vi "Convert_ERDs_Brass.vi"(0 "New Header?":bool, 7 "Array":T7[](array[typedef]) {"ERD Number" format="%.0x"}, 11 "Error In":errorcluster) -> (4 "All_ERD_Data_Bundled_Brass":T1, 15 "Error Out":errorcluster)   [LabVIEW 2016]
doc: "This VI parses the data from ERDs in correct format, units, etc. It handles all hex to dec conversions, hex to enum, and hex to boolean conversions.\n\nIf Raw Data from ERD is blank string, then it will output values from shift register."
uses:
  Common/LabVIEW GEA2 Toolkit/LabVIEW_GEA2_Toolkit.lvlibp/type defs/ERD Read Data Out.ctl
  type defs2/All_Bundled_Data_Brass.ctl
  Laundry Tool 1.0 Support/type defs/Version.ctl
  type defs2/ERD_Always_Show_Brass.ctl
  type defs2/CSV_File_String_Arrays.ctl
  type defs2/Fault Table Array.ctl
  Laundry Tool 1.0 Support/type defs/Fault_Table_Info.ctl
  Common/LabVIEW GEA2 Toolkit/LabVIEW_GEA2_Toolkit.lvlibp
panel:
  # "Software Version"
  # "UI"
  # "MC"
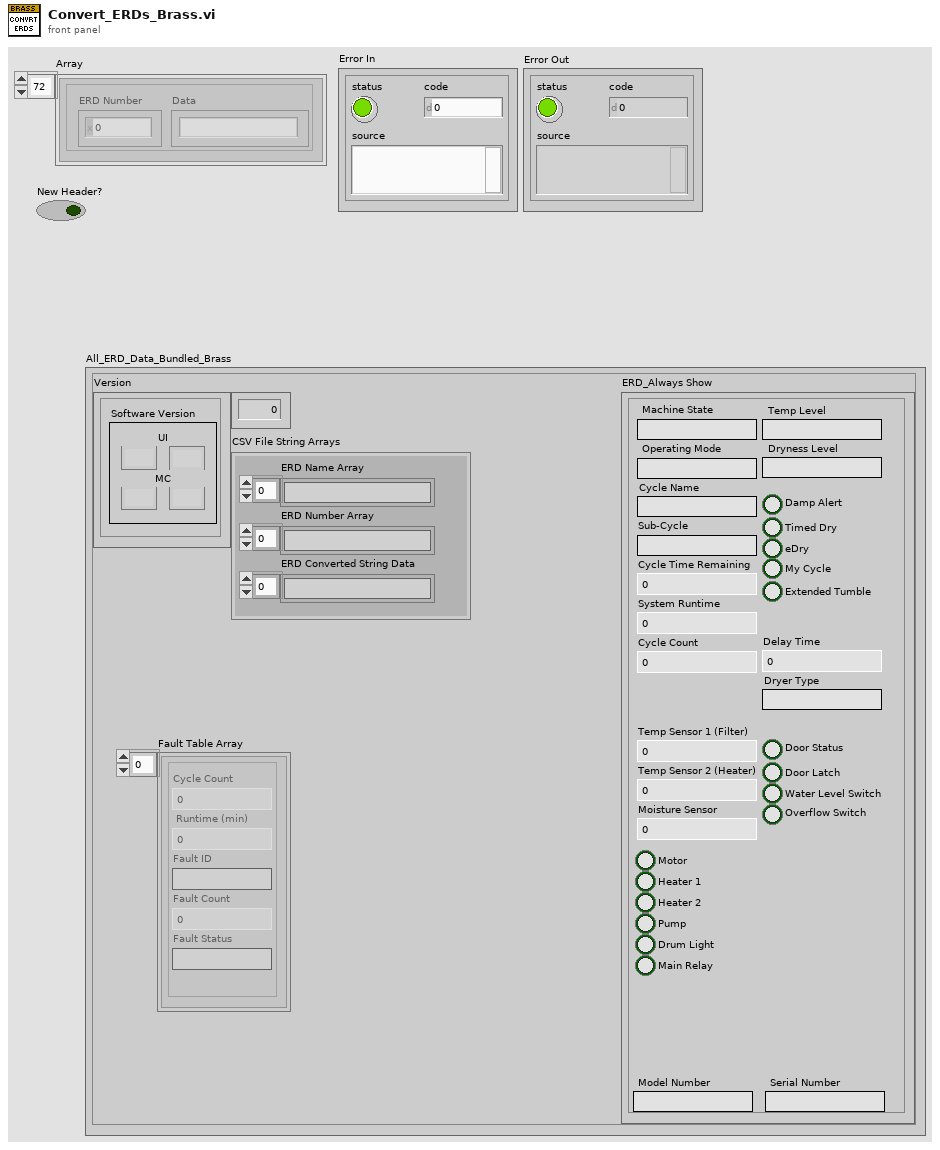
[diagram p1: front panel]
types:
  T1 = typedef "All_Bundled_Data_Brass.ctl" = cluster{"Version":T2, "ERD_Always Show":T3, "Personality Set":u8, "CSV File String Arrays":T4, "Fault Table Array ":T5}
  T2 = typedef "Version.ctl" = cluster{"Critical Major":string, "Critical Minor":string, "Non-Critical Minor":string, "Non-Critical Major":string}
  T3 = typedef "ERD_Always_Show_Brass.ctl" = cluster{"Machine State":string, "Cycle Count":u32, "Dryness Level":string, "Temp Level":string, "Delay Time":u16, "Sub-Cycle":string, "Cycle Name":string, "Model Number":string, "Serial Number":string, "System Runtime":u32, "Cycle Time Remaining":u16, "Operating Mode":string, "Temp Sensor 1 (Filter)":u16, "Water Level Switch":bool, "Overflow Switch":bool, "Door Status":bool, "Door Latch":bool, "Heater 1":bool, "Temp Sensor 2 (Heater)":u16, "Moisture Sensor":u16, "Dryer Type":string, "eDry":bool, "Damp Alert":bool, "Timed Dry":bool, "My Cycle":bool, "Extended Tumble":bool, "Heater 2":bool, "Pump":bool, "Drum Light":bool, "Main Relay":bool, "Motor":bool}
  T4 = typedef "CSV_File_String_Arrays.ctl" = cluster{"ERD Number Array":string[], "ERD Name Array":string[], "ERD Converted String Data":string[]}
  T5 = typedef "Fault Table Array.ctl" = T6[]
  T6 = typedef "Fault_Table_Info.ctl" = cluster{"Cycle Count":u32, " Runtime (min) ":u32, "Fault Status":string, "Fault ID":string, "Fault Count":u16}
  T7 = typedef "LabVIEW_GEA2_Toolkit.lvlibp/ERD Read Data Out.ctl" = cluster{"ERD Number":u16, "Data":string}
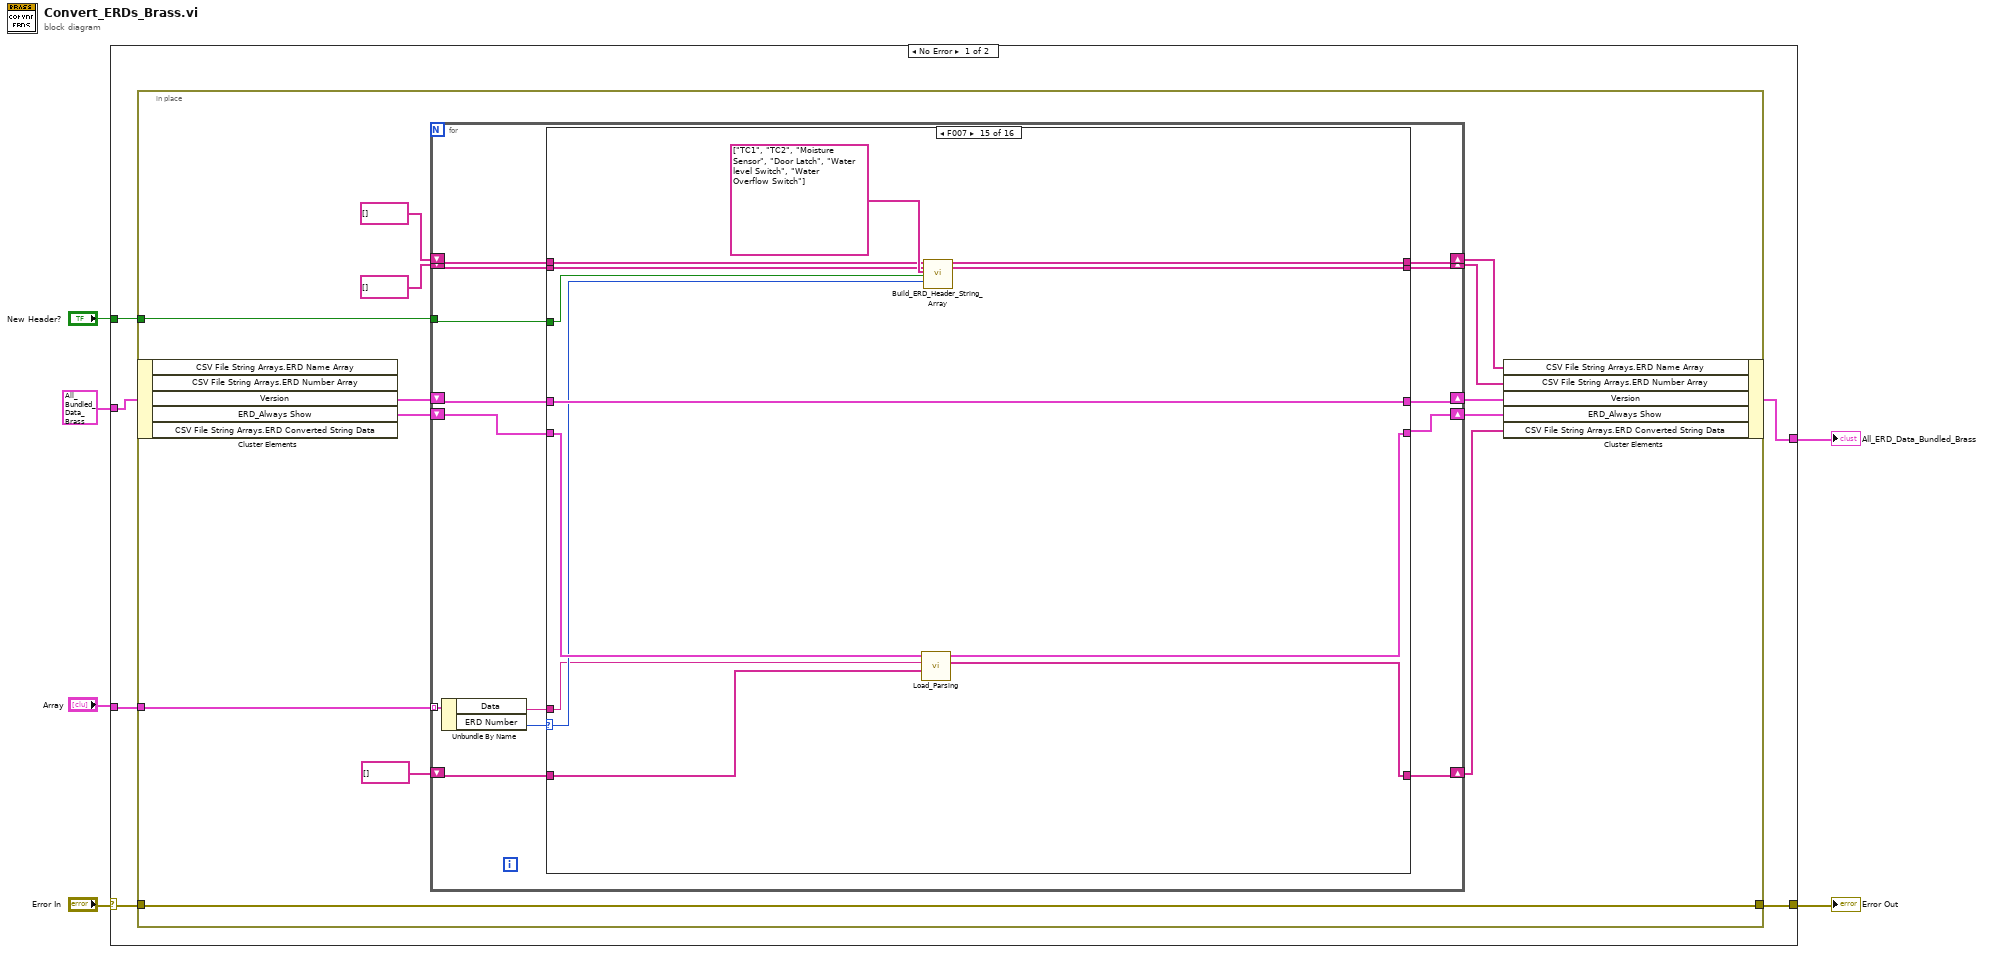
[diagram p0: block diagram]
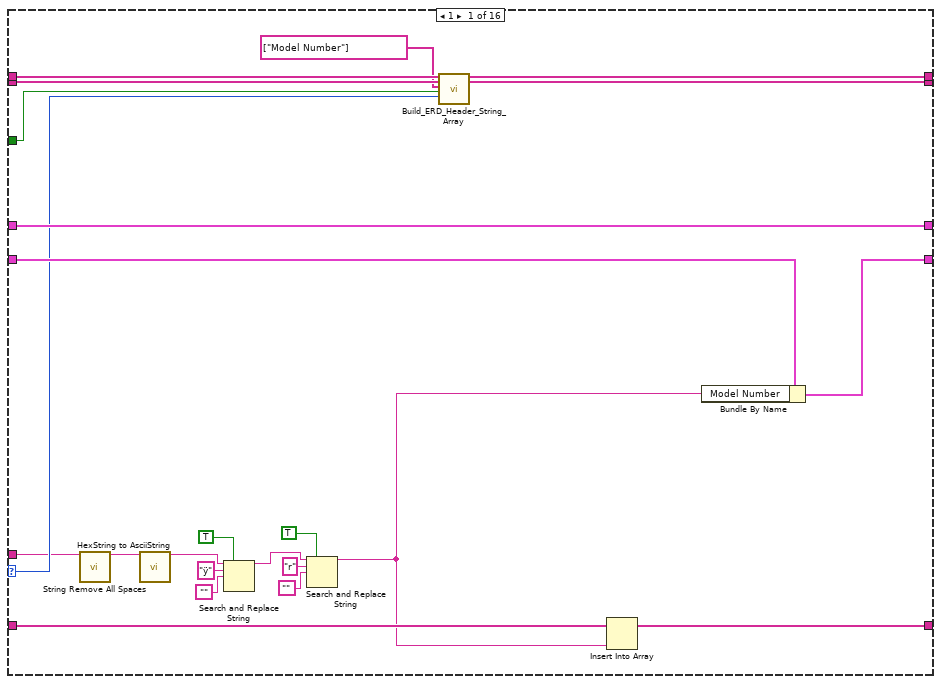
[diagram p2: hidden frame]
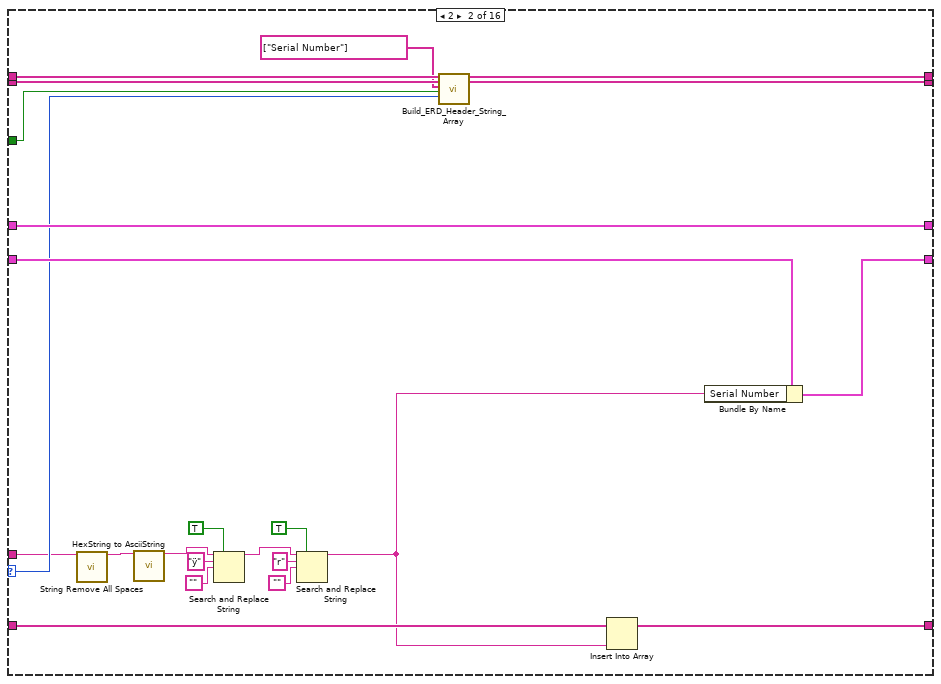
[diagram p3: hidden frame]
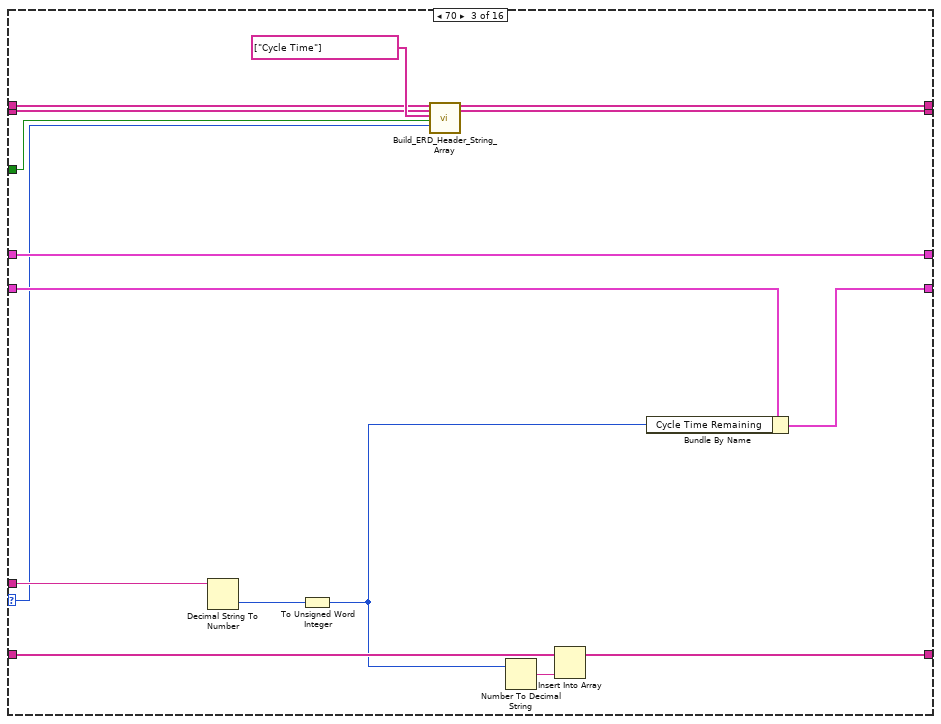
[diagram p4: hidden frame]
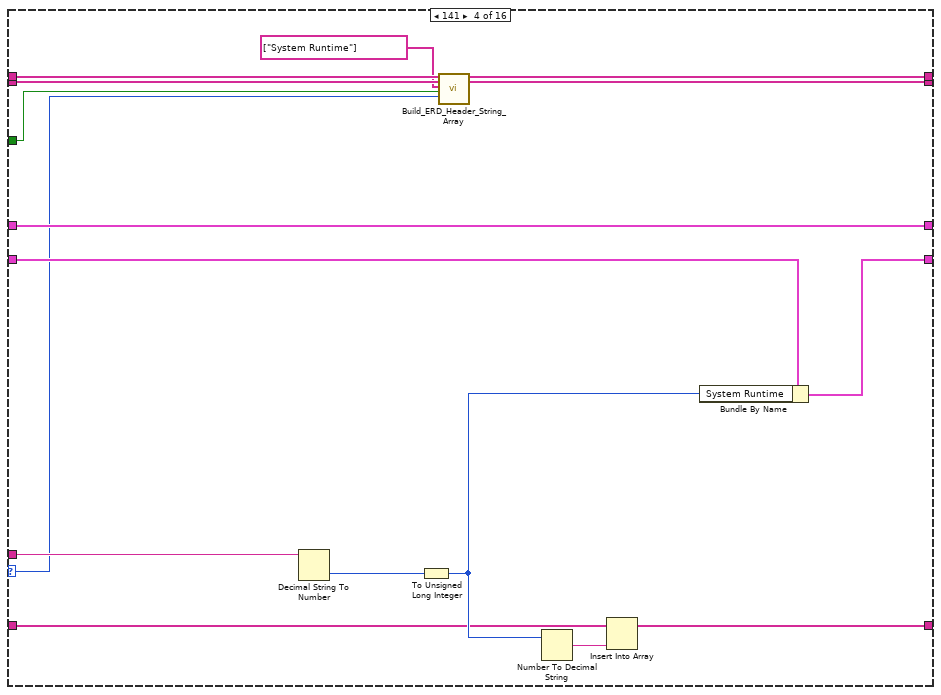
[diagram p5: hidden frame]
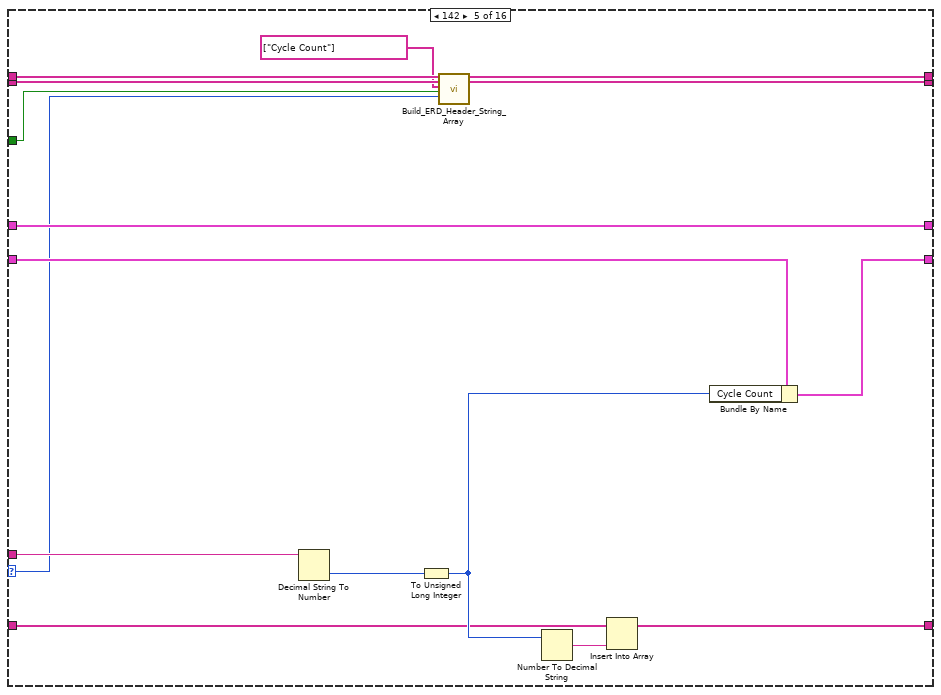
[diagram p6: hidden frame]
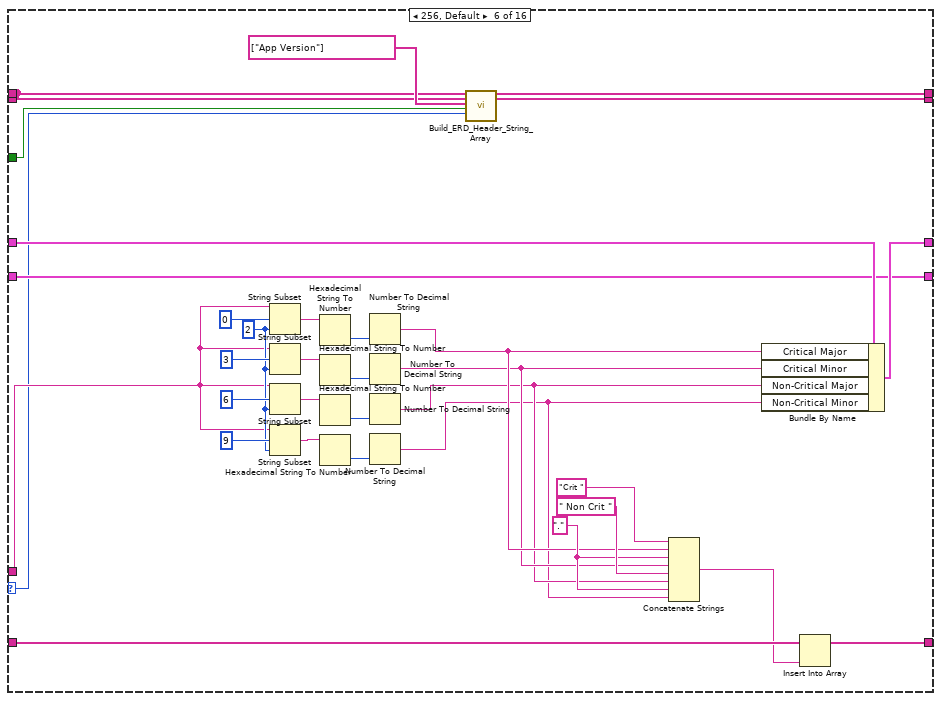
[diagram p7: hidden frame]
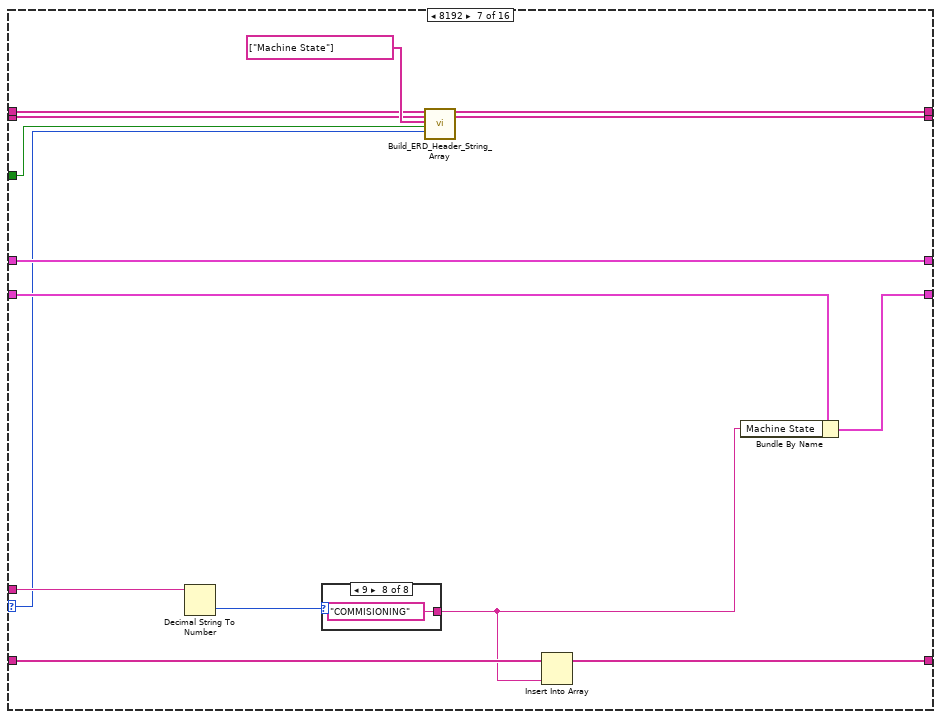
[diagram p8: hidden frame]
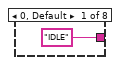
[diagram p9: hidden frame]
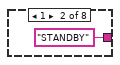
[diagram p10: hidden frame]
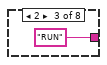
[diagram p11: hidden frame]
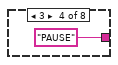
[diagram p12: hidden frame]
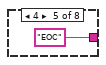
[diagram p13: hidden frame]
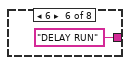
[diagram p14: hidden frame]
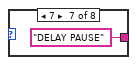
[diagram p15: hidden frame]
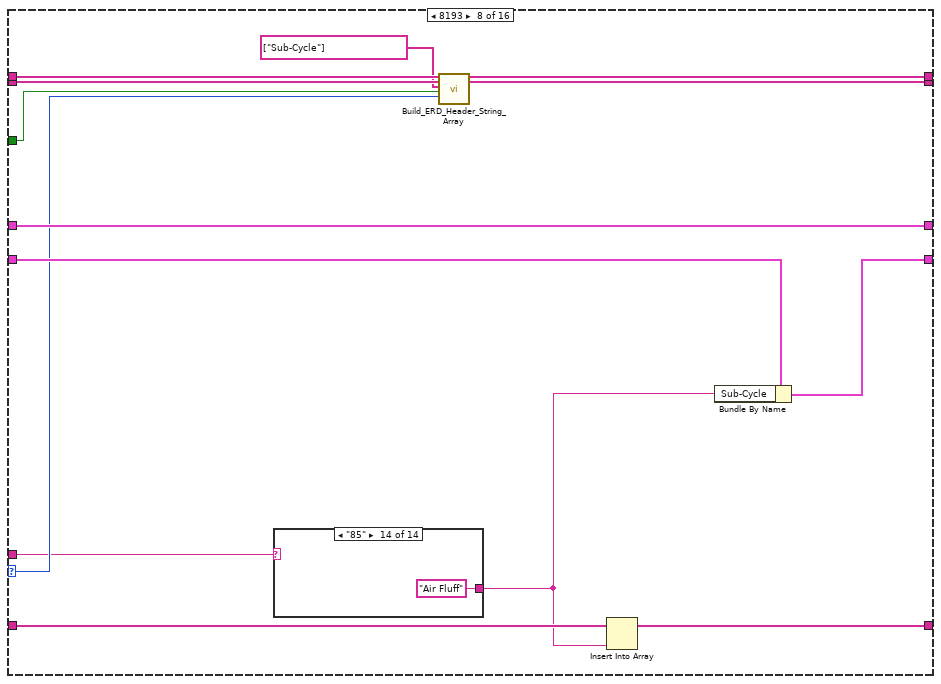
[diagram p16: hidden frame]
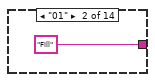
[diagram p18: hidden frame]
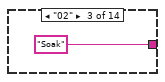
[diagram p19: hidden frame]
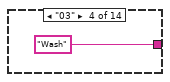
[diagram p20: hidden frame]
diagram:
  n1 = case shown="No Error" "Error In" {
    selector: "Error In" -> [w9 w408]
    tunnel: "Array" -> [w12 _]
    tunnel: [w10 w407] -> w4
    tunnel: T1 {"Version"={"Critical Major"="", "Critical Minor"="", "Non-Critical Minor"="", "Non-Critical Major"=""}, "ERD_Always Show"={"Machine State"="", "Cycle Count"=0, "Dryness Level"="", "Temp Level"="", "Delay Time"=0, "Sub-Cycle"="", "Cycle Name"="", "Model Number"="", "Serial Number"="", "System Runtime"=0, "Cycle Time Remaining"=0, "Operating Mode"="", "Temp Sensor 1 (Filter)"=0, "Water Level Switch"=FALSE, "Overflow Switch"=FALSE, "Door Status"=FALSE, "Door Latch"=FALSE, "Heater 1"=FALSE, "Temp Sensor 2 (Heater)"=0, "Moisture Sensor"=0, "Dryer Type"="", "eDry"=FALSE, "Damp Alert"=FALSE, "Timed Dry"=FALSE, "My Cycle"=FALSE, "Extended Tumble"=FALSE, "Heater 2"=FALSE, "Pump"=FALSE, "Drum Light"=FALSE, "Main Relay"=FALSE, "Motor"=FALSE}, "Personality Set"=0, "CSV File String Arrays"={"ERD Number Array"=[], "ERD Name Array"=[], "ERD Converted String Data"=[]}, "Fault Table Array "=[]} ("ERD_Data_Bundled_Out") -> [w11 w406]
    tunnel: [w8 w406] -> w3
    tunnel: "New Header?" -> [w7 _]
    frame No Error {
      n2 = in-place {
        in-place-border: w12 -> [w25]
        in-place-border: [w22] -> w10
        in-place-border: w9 -> [w22]
        in-place-border: w7 -> [w18]
        n3 = in-place-cluster #1(w11) -> ("Version"=w23:T2, "ERD_Always Show"=w24:T3)  [unwired: 3 out]
        n4 = for {
          tunnel: w25 -> [w39] mode=indexing
          shift-right: [w37] -> w20
          shift-left: w24 -> [w36]
          shift-right: [w34] -> w21
          shift-left: w23 -> [w35]
          shift-right: [w31] -> w13
          shift-left: string[] [] ("ERD String Data") -> [w32]
          tunnel: w18 -> [w30]
          shift-right: [w26] -> w14
          shift-left: string[] [] ("ERD String Data") -> [w29]
          shift-right: [w27] -> w15
          shift-left: string[] [] ("ERD String Data") -> [w28]
          n5 = Unbundle By Name(w39) -> ("Data"=w38:string, "ERD Number"=w33:u16)
          n6 = case shown="F007" w33 {
            selector: w33 -> [w53 w76 w86 w107 w123 w137 w170 w194 w222 w279 w299 w317 w334 w355 w377 w389]
            tunnel: w38 -> [w50 w73 w100 w117 w133 w153 w178 w191 w219 w276 w313 w327 w345 w366 w376 w400]
            tunnel: [w61 w84 w98 w115 w131 w150 w181 w202 w230 w287 w311 w328 w346 w367 w387 w401] -> w37
            tunnel: w36 -> [w62 w85 w99 w116 w132 w150 w180 w203 w231 w288 w312 w329 w347 w368 w388 w402]
            tunnel: w35 -> [w60 w83 w97 w114 w130 w152 w177 w201 w229 w286 w310 w326 w344 w365 w386 w399]
            tunnel: [w60 w83 w97 w114 w130 w151 w177 w201 w229 w286 w310 w326 w344 w365 w386 w399] -> w34
            tunnel: w32 -> [w58 w81 w90 w112 w128 _ w174 w199 w227 w284 w303 w321 w338 w359 w381 w393]
            tunnel: [w56 w79 w88 w110 w126 w139 w172 w197 w225 w282 w301 w319 w336 w357 w379 w391] -> w31
            tunnel: w30 -> [w54 w77 w87 w108 w124 w138 w171 w195 w223 w280 w300 w318 w335 w356 w378 w390]
            tunnel: w29 -> [w59 w82 w91 w113 w129 w141 w175 w200 w228 w285 w304 w322 w339 w360 w382 w394]
            tunnel: w28 -> [w52 w75 w95 w103 w119 w144 w169 w193 w221 w278 w308 w325 w343 w364 w385 w398]
            tunnel: [w51 w74 w94 w102 w118 w143 w168 w192 w220 w277 w307 w324 w342 w363 w384 w397] -> w27
            tunnel: [w57 w80 w89 w111 w127 w140 w173 w198 w226 w283 w302 w320 w337 w358 w380 w392] -> w26
            frame 1 {
              n7 = call "String Remove All Spaces.vi"("Input String"=w50) -> ("Spaces Removed"=w49:string)  [unwired: 13 in, 1 out]
              n8 = call "HexString to AsciiString.vi"("Hex String"=w49) -> ("ASCII String"=w45:string)  [unwired: 13 in, 1 out]
              n9 = Search and Replace String(replace all?=TRUE ("replace all? (F)"), input string=w45, search string="ÿ", replace string="") -> (result string=w41:string)  [unwired: 4 in, 3 out]
              n10 = Search and Replace String(replace all?=TRUE ("replace all? (F)"), input string=w41, search string="r", replace string="") -> (result string=w44:string)  [unwired: 4 in, 3 out]
              n11 = call "Build_ERD_Header_String_Array.vi"("ERD Name Array In"=w59, "ERD Number Array In"=w58, "ERD Name List"=string[] ["Model Number"], "New Header?"=w54, "ERD Number"=w53) -> ("ERD Name Array Out"=w57:string[], "ERD Number Array Out"=w56:string[])  [unwired: 13 in]
              n12 = Insert Into Array(array=w52, new element=w44) -> (w51:string[])  [unwired: 1 in]
              n13 = Bundle By Name(cluster=w62, "Model Number"=w44) -> (w61:T3)
            }
            frame 2 {
              n14 = call "String Remove All Spaces.vi"("Input String"=w73) -> ("Spaces Removed"=w72:string)  [unwired: 13 in, 1 out]
              n15 = call "HexString to AsciiString.vi"("Hex String"=w72) -> ("ASCII String"=w69:string)  [unwired: 13 in, 1 out]
              n16 = Search and Replace String(replace all?=TRUE ("replace all? (F)"), input string=w69, search string="ÿ", replace string="") -> (result string=w64:string)  [unwired: 4 in, 3 out]
              n17 = Search and Replace String(replace all?=TRUE ("replace all? (F)"), input string=w64, search string="r", replace string="") -> (result string=w63:string)  [unwired: 4 in, 3 out]
              n18 = call "Build_ERD_Header_String_Array.vi"("ERD Name Array In"=w82, "ERD Number Array In"=w81, "ERD Name List"=string[] ["Serial Number"], "New Header?"=w77, "ERD Number"=w76) -> ("ERD Name Array Out"=w80:string[], "ERD Number Array Out"=w79:string[])  [unwired: 13 in]
              n19 = Insert Into Array(array=w75, new element=w63) -> (w74:string[])  [unwired: 1 in]
              n20 = Bundle By Name(cluster=w85, "Serial Number"=w63) -> (w84:T3)
            }
            frame 70 {
              n21 = Decimal String To Number(string=w100) -> (number=w101:i32)  [unwired: 2 in, 1 out]
              n22 = To Unsigned Word Integer(number=w101) -> (unsigned 16bit integer=w93:u16)
              n23 = call "Build_ERD_Header_String_Array.vi"("ERD Name Array In"=w91, "ERD Number Array In"=w90, "ERD Name List"=string[] ["Cycle Time"], "New Header?"=w87, "ERD Number"=w86) -> ("ERD Name Array Out"=w89:string[], "ERD Number Array Out"=w88:string[])  [unwired: 13 in]
              n24 = Number To Decimal String(number=w93) -> (decimal integer string=w96:string)  [unwired: 1 in]
              n25 = Insert Into Array(array=w95, new element=w96) -> (w94:string[])  [unwired: 1 in]
              n26 = Bundle By Name(cluster=w99, "Cycle Time Remaining"=w93) -> (w98:T3)
            }
            frame 141 {
              n27 = Decimal String To Number(string=w117) -> (number=w105:i32)  [unwired: 2 in, 1 out]
              n28 = To Unsigned Long Integer(number=w105) -> (unsigned 32bit integer=w104:u32)
              n29 = call "Build_ERD_Header_String_Array.vi"("ERD Name Array In"=w113, "ERD Number Array In"=w112, "ERD Name List"=string[] ["System Runtime"], "New Header?"=w108, "ERD Number"=w107) -> ("ERD Name Array Out"=w111:string[], "ERD Number Array Out"=w110:string[])  [unwired: 13 in]
              n30 = Number To Decimal String(number=w104) -> (decimal integer string=w106:string)  [unwired: 1 in]
              n31 = Insert Into Array(array=w103, new element=w106) -> (w102:string[])  [unwired: 1 in]
              n32 = Bundle By Name(cluster=w116, "System Runtime"=w104) -> (w115:T3)
            }
            frame 142 {
              n33 = Decimal String To Number(string=w133) -> (number=w121:i32)  [unwired: 2 in, 1 out]
              n34 = To Unsigned Long Integer(number=w121) -> (unsigned 32bit integer=w120:u32)
              n35 = call "Build_ERD_Header_String_Array.vi"("ERD Name Array In"=w129, "ERD Number Array In"=w128, "ERD Name List"=string[] ["Cycle Count"], "New Header?"=w124, "ERD Number"=w123) -> ("ERD Name Array Out"=w127:string[], "ERD Number Array Out"=w126:string[])  [unwired: 13 in]
              n36 = Number To Decimal String(number=w120) -> (decimal integer string=w122:string)  [unwired: 1 in]
              n37 = Insert Into Array(array=w119, new element=w122) -> (w118:string[])  [unwired: 1 in]
              n38 = Bundle By Name(cluster=w132, "Cycle Count"=w120) -> (w131:T3)
            }
            frame 256, Default {
              w147 = "." ("element")
              w154 = 2 ("length (rest)")
              n39 = String Subset(string=w153, offset (0)=0 ("length (rest)"), length (rest)=w154) -> (substring=w166:string)
              n40 = String Subset(string=w153, offset (0)=3 ("length (rest)"), length (rest)=w154) -> (substring=w162:string)
              n41 = String Subset(string=w153, offset (0)=6 ("length (rest)"), length (rest)=w154) -> (substring=w157:string)
              n42 = String Subset(string=w153, offset (0)=9 ("length (rest)"), length (rest)=w154) -> (substring=w156:string)
              n43 = Hexadecimal String To Number(string=w166) -> (number=w161:u32)  [unwired: 2 in, 1 out]
              n44 = Hexadecimal String To Number(string=w162) -> (number=w160:u32)  [unwired: 2 in, 1 out]
              n45 = Hexadecimal String To Number(string=w157) -> (number=w159:u32)  [unwired: 2 in, 1 out]
              n46 = Hexadecimal String To Number(string=w156) -> (number=w158:u32)  [unwired: 2 in, 1 out]
              n47 = Number To Decimal String(number=w161) -> (decimal integer string=w146:string)  [unwired: 1 in]
              n48 = Number To Decimal String(number=w160) -> (decimal integer string=w145:string)  [unwired: 1 in]
              n49 = Number To Decimal String(number=w159) -> (decimal integer string=w136:string)  [unwired: 1 in]
              n50 = Number To Decimal String(number=w158) -> (decimal integer string=w135:string)  [unwired: 1 in]
              n51 = call "Build_ERD_Header_String_Array.vi"("ERD Name Array In"=w141, "ERD Number Array In"=w141, "ERD Name List"=string[] ["App Version"], "New Header?"=w138, "ERD Number"=w137) -> ("ERD Name Array Out"=w140:string[], "ERD Number Array Out"=w139:string[])  [unwired: 13 in]
              n52 = Concatenate Strings("Crit " ("element"), w146, w147, w145, " Non Crit " ("element"), w136, w147, w135) -> (w134:string)
              n53 = Bundle By Name(cluster=w152, "Critical Major"=w146, "Critical Minor"=w145, "Non-Critical Major"=w136, "Non-Critical Minor"=w135) -> (w151:T2)
              n54 = Insert Into Array(array=w144, new element=w134) -> (w143:string[])  [unwired: 1 in]
            }
            frame 8192 {
              n55 = Decimal String To Number(string=w178) -> (number=w179:i32)  [unwired: 2 in, 1 out]
              n56 = case shown="9" w179 {
                tunnel: ["IDLE" "STANDBY" "RUN" "PAUSE" "EOC" "DELAY RUN" "DELAY PAUSE" "COMMISIONING"] -> w167
                frame 0, Default {
                }
                frame 1 {
                }
                frame 2 {
                }
                frame 3 {
                }
                frame 4 {
                }
                frame 6 {
                }
                frame 7 {
                }
                frame 9 {
                }
              }
              n57 = call "Build_ERD_Header_String_Array.vi"("ERD Name Array In"=w175, "ERD Number Array In"=w174, "ERD Name List"=string[] ["Machine State"], "New Header?"=w171, "ERD Number"=w170) -> ("ERD Name Array Out"=w173:string[], "ERD Number Array Out"=w172:string[])  [unwired: 13 in]
              n58 = Insert Into Array(array=w169, new element=w167) -> (w168:string[])  [unwired: 1 in]
              n59 = Bundle By Name(cluster=w180, "Machine State"=w167) -> (w181:T3)
            }
            frame 8193 {
              n60 = case shown="\"85\"" w191 {
                selector: w191 -> [w204 _ _ _ _ _ _ _ _ _ _ _ _ _]
                tunnel: [w204 "Fill" "Soak" "Wash" "Rinse" "Spin" "Tumble" "Load Size Detection" "Drying" "Mist/Steam" "Cool Down" "Extnd Tumble" "Damp" "Air Fluff"] -> w190
                frame "00", Default {
                }
                frame "01" {
                }
                frame "02" {
                }
                frame "03" {
                }
                frame "04" {
                }
                frame "05" {
                }
                frame "09" {
                }
                frame "0A" {
                }
                frame "80" {
                }
                frame "81" {
                }
                frame "82" {
                }
                frame "83" {
                }
                frame "84" {
                }
                frame "85" {
                }
              }
              n61 = call "Build_ERD_Header_String_Array.vi"("ERD Name Array In"=w200, "ERD Number Array In"=w199, "ERD Name List"=string[] ["Sub-Cycle"], "New Header?"=w195, "ERD Number"=w194) -> ("ERD Name Array Out"=w198:string[], "ERD Number Array Out"=w197:string[])  [unwired: 13 in]
              n62 = Insert Into Array(array=w193, new element=w190) -> (w192:string[])  [unwired: 1 in]
              n63 = Bundle By Name(cluster=w203, "Sub-Cycle"=w190) -> (w202:T3)
            }
            frame 8202 {
              n64 = case shown="\"90\"" w219 {
                tunnel: ["Not Defined" "Basket Clean" "Drain & Spin" "Quick Rinse" "Bulky Items" "Sanitize" "Towels & Sheets" "Steam Refresh" "Normal/Mixed" "Whites" "Dark Colors" "Jeans" "Hand Wash" "Delicates" "Speed Wash" "Heavy Duty" "Allergen" "Power Clean" "Rinse & Spin" "Single Item" "Colors" "Cold Wash" "Water on Demand" "Tub Clean" "Casuals with Steam" "Stain Wash with Steam" "Cottons" "Easy Care" "Active Wear" "Timed Dry" "Dewrinkle" "Air Fluff" "Steam Refresh" "Steam Dewrinkle" "Speed Dry" "Mixed" "Quick Dry" "Casuals" "Warm Up" "Energy Saver" "Anitbacterial" "Rack Dry" "Baby Care"] -> w218
                frame "00", Default {
                }
                frame "01" {
                }
                frame "02" {
                }
                frame "03" {
                }
                frame "04" {
                }
                frame "05" {
                }
                frame "06" {
                }
                frame "07" {
                }
                frame "08" {
                }
                frame "09" {
                }
                frame "0A" {
                }
                frame "0B" {
                }
                frame "0C" {
                }
                frame "0D" {
                }
                frame "0E" {
                }
                frame "0F" {
                }
                frame "10" {
                }
                frame "11" {
                }
                frame "12" {
                }
                frame "13" {
                }
                frame "14" {
                }
                frame "15" {
                }
                frame "16" {
                }
                frame "17" {
                }
                frame "18" {
                }
                frame "19" {
                }
                frame "80" {
                }
                frame "81" {
                }
                frame "82" {
                }
                frame "83" {
                }
                frame "84" {
                }
                frame "85" {
                }
                frame "86" {
                }
                frame "87" {
                }
                frame "88" {
                }
                frame "89" {
                }
                frame "8A" {
                }
                frame "8B" {
                }
                frame "8C" {
                }
                frame "8D" {
                }
                frame "8E" {
                }
                frame "8F" {
                }
                frame "90" {
                }
              }
              n65 = call "Build_ERD_Header_String_Array.vi"("ERD Name Array In"=w228, "ERD Number Array In"=w227, "ERD Name List"=string[] ["Cycle Name"], "New Header?"=w223, "ERD Number"=w222) -> ("ERD Name Array Out"=w226:string[], "ERD Number Array Out"=w225:string[])  [unwired: 13 in]
              n66 = Insert Into Array(array=w221, new element=w218) -> (w220:string[])  [unwired: 1 in]
              n67 = Bundle By Name(cluster=w231, "Cycle Name"=w218) -> (w230:T3)
            }
            frame 8206 {
              n68 = case shown="\"09\"" w276 {
                tunnel: ["Consumer Mode" "Service Mode" "factory/EOL Mode" "Continuous Cycle Mode" "Rapid Relay Mode" "FCT Mode" "Model Plug" "Demo Mode" "Consumer Error Mode" "Floor Type Selection Mode"] -> w275
                frame "00", Default {
                }
                frame "01" {
                }
                frame "02" {
                }
                frame "03" {
                }
                frame "04" {
                }
                frame "05" {
                }
                frame "06" {
                }
                frame "07" {
                }
                frame "08" {
                }
                frame "09" {
                }
              }
              n69 = call "Build_ERD_Header_String_Array.vi"("ERD Name Array In"=w285, "ERD Number Array In"=w284, "ERD Name List"=string[] ["Operating Mode"], "New Header?"=w280, "ERD Number"=w279) -> ("ERD Name Array Out"=w283:string[], "ERD Number Array Out"=w282:string[])  [unwired: 13 in]
              n70 = Insert Into Array(array=w278, new element=w275) -> (w277:string[])  [unwired: 1 in]
              n71 = Bundle By Name(cluster=w288, "Operating Mode"=w275) -> (w287:T3)
            }
            frame 8208 {
              n72 = Decimal String To Number(string=w313) -> (number=w314:i32)  [unwired: 2 in, 1 out]
              n73 = To Unsigned Word Integer(number=w314) -> (unsigned 16bit integer=w306:u16)
              n74 = call "Build_ERD_Header_String_Array.vi"("ERD Name Array In"=w304, "ERD Number Array In"=w303, "ERD Name List"=string[] ["Delay Time"], "New Header?"=w300, "ERD Number"=w299) -> ("ERD Name Array Out"=w302:string[], "ERD Number Array Out"=w301:string[])  [unwired: 13 in]
              n75 = Number To Decimal String(number=w306) -> (decimal integer string=w309:string)  [unwired: 1 in]
              n76 = Insert Into Array(array=w308, new element=w309) -> (w307:string[])  [unwired: 1 in]
              n77 = Bundle By Name(cluster=w312, "Delay Time"=w306) -> (w311:T3)
            }
            frame 8210 {
              n78 = case shown="\"01\"" w327 {
                tunnel: ["Open" "Closed"] -> w315
                tunnel: [FALSE TRUE] -> w316
                frame "00", Default {
                }
                frame "01" {
                }
              }
              n79 = call "Build_ERD_Header_String_Array.vi"("ERD Name Array In"=w322, "ERD Number Array In"=w321, "ERD Name List"=string[] ["Door Status"], "New Header?"=w318, "ERD Number"=w317) -> ("ERD Name Array Out"=w320:string[], "ERD Number Array Out"=w319:string[])  [unwired: 13 in]
              n80 = Insert Into Array(array=w325, new element=w315) -> (w324:string[])  [unwired: 1 in]
              n81 = Bundle By Name(cluster=w329, "Door Status"=w316) -> (w328:T3)
            }
            frame 8217 {
              n82 = case shown="Default" w345 {
                selector: w345 -> [w348 _ _ _ _ _ _]
                tunnel: [w348 "No Heat" "Extra Low" "Low" "Medium" "High" "Disable"] -> w341
                frame Default {
                }
                frame "00" {
                }
                frame "01" {
                }
                frame "02" {
                }
                frame "03" {
                }
                frame "04" {
                }
                frame "5" {
                }
              }
              n83 = call "Build_ERD_Header_String_Array.vi"("ERD Name Array In"=w339, "ERD Number Array In"=w338, "ERD Name List"=string[] ["Temp Level"], "New Header?"=w335, "ERD Number"=w334) -> ("ERD Name Array Out"=w337:string[], "ERD Number Array Out"=w336:string[])  [unwired: 13 in]
              n84 = Insert Into Array(array=w343, new element=w341) -> (w342:string[])  [unwired: 1 in]
              n85 = Bundle By Name(cluster=w347, "Temp Level"=w341) -> (w346:T3)
            }
            frame 8218 {
              n86 = case shown="\"05\"" w366 {
                selector: w366 -> [w369 _ _ _ _ _ _]
                tunnel: [w369 "Damp" "Less Dry" "Dry" "More Dry" "Extra Dry" "N/A"] -> w362
                frame Default {
                }
                frame "00" {
                }
                frame "01" {
                }
                frame "02" {
                }
                frame "03" {
                }
                frame "04" {
                }
                frame "05" {
                }
              }
              n87 = call "Build_ERD_Header_String_Array.vi"("ERD Name Array In"=w360, "ERD Number Array In"=w359, "ERD Name List"=string[] ["Dryness Level"], "New Header?"=w356, "ERD Number"=w355) -> ("ERD Name Array Out"=w358:string[], "ERD Number Array Out"=w357:string[])  [unwired: 13 in]
              n88 = Insert Into Array(array=w364, new element=w362) -> (w363:string[])  [unwired: 1 in]
              n89 = Bundle By Name(cluster=w368, "Dryness Level"=w362) -> (w367:T3)
            }
            frame 61447 {
              n90 = call "Load_Parsing.vi"("ERD String Data in"=w385, "Data"=w376, "ERD_Always Show in"=w388) -> ("ERD String Data out"=w384:string[], "ERD_Always Show out"=w387:T3)  [unwired: 7 in]
              n91 = call "Build_ERD_Header_String_Array.vi"("ERD Name Array In"=w382, "ERD Number Array In"=w381, "ERD Name List"=string[] ["TC1", "TC2", "Moisture Sensor", "Door Latch", "Water level Switch", "Water Overflow Switch"], "New Header?"=w378, "ERD Number"=w377) -> ("ERD Name Array Out"=w380:string[], "ERD Number Array Out"=w379:string[])  [unwired: 13 in]
            }
            frame 61448 {
              n92 = case shown="\"01\"" w400 {
                selector: w400 -> [w403 _ _]
                tunnel: [w403 "Condenser" "Vented"] -> w396
                frame Default {
                }
                frame "00" {
                }
                frame "01" {
                }
              }
              n93 = call "Build_ERD_Header_String_Array.vi"("ERD Name Array In"=w394, "ERD Number Array In"=w393, "ERD Name List"=string[] ["Dryer Type"], "New Header?"=w390, "ERD Number"=w389) -> ("ERD Name Array Out"=w392:string[], "ERD Number Array Out"=w391:string[])  [unwired: 13 in]
              n94 = Insert Into Array(array=w398, new element=w396) -> (w397:string[])  [unwired: 1 in]
              n95 = Bundle By Name(cluster=w402, "Dryer Type"=w396) -> (w401:T3)
            }
          }
        }
        n96 = in-place-cluster #1("CSV File String Arrays.ERD Name Array"=w14, "CSV File String Arrays.ERD Number Array"=w13, "Version"=w21, "ERD_Always Show"=w20, "CSV File String Arrays.ERD Converted String Data"=w15) -> (w8:T1)
      }
    }
    frame Error {
      n97 = Unbundle By Name(w408) -> ("code"=w412:i32, "status"=w413:bool, "source"=w410:string)
      n98 = Equal?(x=w412, y=-5006) -> (x = y?=w416:bool)
      n99 = case shown="True" w416 {
        tunnel: [w420 FALSE] -> w414
        tunnel: w413 -> [w420 _]
        tunnel: w412 -> [w419 w422]
        tunnel: [w419 w422] -> w411
        tunnel: [w418 w421] -> w409
        tunnel: w410 -> [w418 w421]
        frame False {
        }
        frame True {
        }
      }
      n100 = Bundle By Name(cluster=errorcluster {"status"=FALSE, "code"=0, "source"=""} ("error constant"), "status"=w414, "code"=w411, "source"=w409) -> (w407:errorcluster)
    }
  }
  "Error Out" <- w4
  "All_ERD_Data_Bundled_Brass" <- w3
